vi "event_generate_auth.vi"(8 "error in (no error)":errorcluster, 10 "state":string, 11 "code":string) -> ()   [LabVIEW 2015, in "lv-dropbox.lvlib" / "examples.lvlib"]
uses:
  examples.lvlib
  private/_controls/authorization_response.ctl
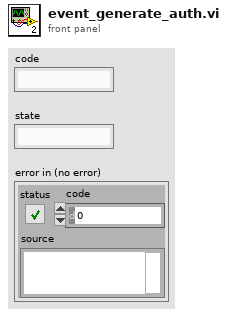
[diagram p1: front panel]
types:
  T1 = typedef "lv-dropbox.lvlib/examples.lvlib/authorization_response.ctl" = cluster{"code":string, "state":string}
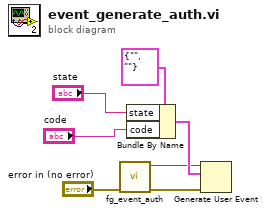
[diagram p0: block diagram]
diagram:
  n1 = call "fg_event_auth.vi"("error in (no error)"="error in (no error)") -> ("error out"=w2:errorcluster, "auth"=w1:refnum<user-event>)  [unwired: 9 in]
  n2 = Bundle By Name(cluster=T1 {"code"="", "state"=""} ("event data"), "state"="state", "code"="code") -> (w4:T1)
  n3 = Generate User Event(user event=w1, event data cluster=w4, error in=w2) -> ()  [unwired: 1 in, 2 out]
